vi "AIT 1553 - Write Parameters.vi"(0 "File Path":path, 5 "Bus In":T1, 11 "error in (no error)":errorcluster) -> (15 "error out":errorcluster)   [LabVIEW 2013]
uses:
  Controls/1553_Bus.ctl
  Controls/1553_Bus_Controller.ctl
  Controls/1553_BC_Message.ctl
  Controls/664 -Param.ctl
  Controls/1553_Acyclic_Frame.ctl
  Controls/1553_Bus_Monitor.ctl
  Controls/1553_BM_Message.ctl
  Controls/1553_RT_Message.ctl
  <vilib>/NI/GXML/GXML.lvlib
  AIT 664 Custom Device.lvlib
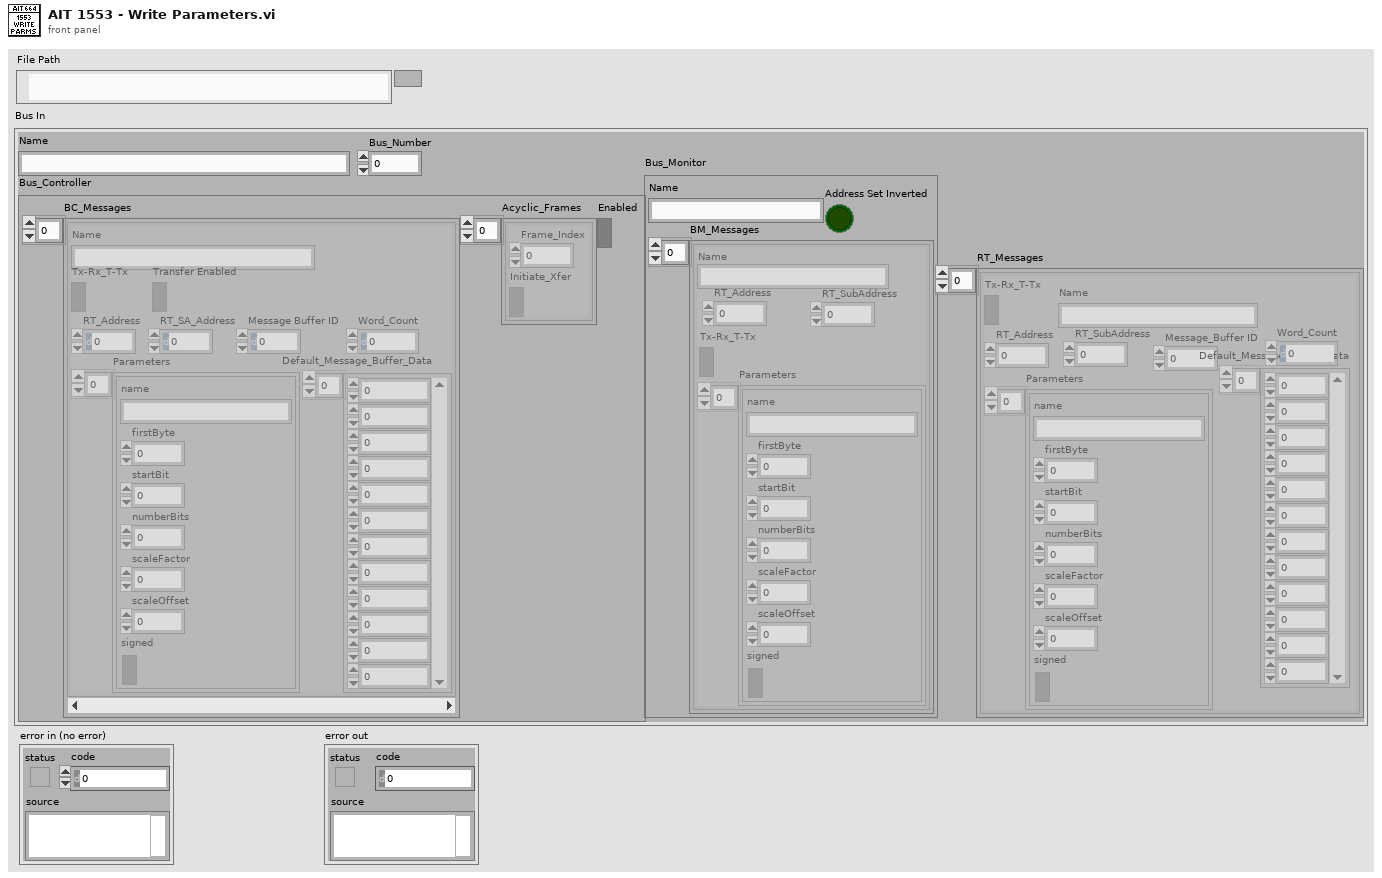
[diagram p1: front panel]
types:
  T1 = typedef "AIT 664 Custom Device.lvlib/1553_Bus.ctl" = cluster{"Name":string, "Bus_Number":u8, "Bus_Controller":T2, "Bus_Monitor":T6, "RT_Messages":T8[]}
  T2 = typedef "AIT 664 Custom Device.lvlib/1553_Bus_Controller.ctl" = cluster{"BC_Messages":T3[], "Acyclic_Frames":T5[], "Enabled":bool}
  T3 = typedef "AIT 664 Custom Device.lvlib/1553_BC_Message.ctl" = cluster{"Name":string, "Tx-Rx_T-Tx":bool, "RT_Address":u8, "RT_SA_Address":u8, "Parameters":T4[], "Transfer Enabled":bool, "Message Buffer ID":u16, "Default_Message_Buffer_Data":u16[], "Word_Count":u8}
  T4 = typedef "AIT 664 Custom Device.lvlib/664 -Param.ctl" = cluster{"name":string, "firstByte":i32, "startBit":i32, "numberBits":i32, "scaleFactor":dbl, "scaleOffset":dbl, "signed":bool}
  T5 = typedef "AIT 664 Custom Device.lvlib/1553_Acyclic_Frame.ctl" = cluster{"Frame_Index":u8, "Initiate_Xfer":bool}
  T6 = typedef "AIT 664 Custom Device.lvlib/1553_Bus_Monitor.ctl" = cluster{"Name":string, "BM_Messages":T7[], "Address Set Inverted":bool}
  T7 = typedef "AIT 664 Custom Device.lvlib/1553_BM_Message.ctl" = cluster{"RT_Address":u8, "RT_SubAddress":u8, "Tx-Rx_T-Tx":bool, "Parameters":T4[], "Name":string}
  T8 = typedef "AIT 664 Custom Device.lvlib/1553_RT_Message.ctl" = cluster{"RT_Address":u8, "RT_SubAddress":u8, "Tx-Rx_T-Tx":bool, "Parameters":T4[], "Message_Buffer ID":u16, "Default_Message_Buffer_Data":u16[], "Word_Count":u8, "Name":string}
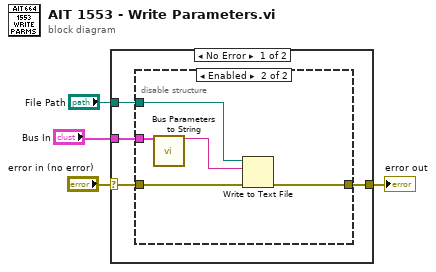
[diagram p0: block diagram]
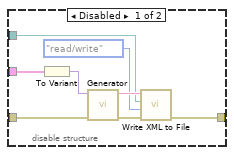
[diagram p2: hidden frame]
diagram:
  n1 = case shown="No Error" "error in (no error)" {
    selector: "error in (no error)" -> [w8 w22]
    tunnel: [w6 w22] -> w3
    tunnel: "Bus In" -> [w7 _]
    tunnel: "File Path" -> [w5 _]
    frame No Error {
      n2 = disable-structure shown="Enabled" {
        disable-tunnel: w8 -> [w15 w19]
        disable-tunnel: w7 -> [w14 w21]
        disable-tunnel: [w12 w18] -> w6
        disable-tunnel: w5 -> [w9 w20]
        frame Disabled {
          n3 = To Variant(anything=w14) -> (Variant=w16:variant)
          n4 = call <vilib>:"Generator.vi"("error in"=w15, "Variant"=w16) -> ("error out"=w13:errorcluster, "XML String Out"=w11:string)  [unwired: 8 in]
          n5 = call <vilib>:"Write XML to File.vi"("error in"=w13, "file access"=enum16{"read/write", "read-only", "write-only"}."read/write", "XML File Path"=w9, "XML Input"=w11) -> ("error out"=w12:errorcluster)  [unwired: 7 in]
        }
        frame Enabled {
          n6 = call "Bus Parameters to String.vi"("Bus"=w21) -> ("Parms List"=w17:string)  [unwired: 14 in]
          n7 = Write to Text File(file (use dialog)=w20, text=w17, error in=w19) -> (error out=w18:errorcluster)  [unwired: 1 in, 2 out]
        }
      }
    }
    frame Error {
    }
  }
  "error out" <- w3
